vi "FrequencyToMilliseconds.vi"(11 "Frequency":dbl) -> (3 "Numeric":i64)   [LabVIEW 2018]
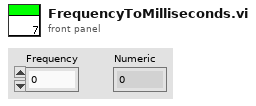
[diagram p1: front panel]
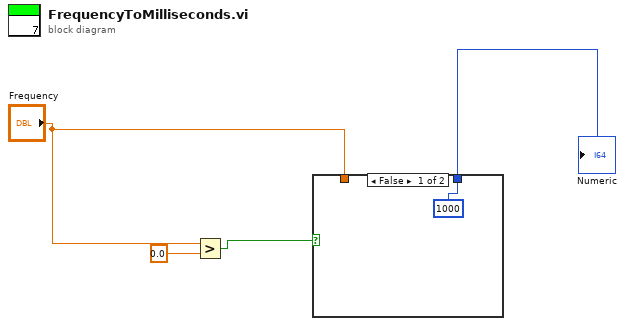
[diagram p0: block diagram]
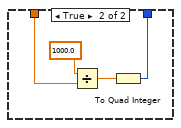
[diagram p2: hidden frame]
diagram:
  n1 = Greater?(x="Frequency", y=0.0) -> (0:w3:bool)
  n2 = case shown="False" w3 {
    tunnel: [i64 1000 w8] -> w2
    tunnel: "Frequency" -> [_ w7]
    frame False {
    }
    frame True {
      n3 = Divide(x=1000.0, y=w7) -> (x/y=w9:dbl)
      n4 = To Quad Integer(1:w9) -> (0:w8:i64)
    }
  }
  "Numeric" <- w2
